vi "FisherPaykel Stop Motor.vi"(0 "VISA Refnum in":refnum<visa-resource-name>, 1 "Debug":bool, 2 "Use GEA Inverter Output":bool, 5 "Main Command":T2=">STP", 7 "GEA2 Reference In":refnum<k24>, 11 "Error In":errorcluster, 12 "GEA Stop Toggle":u8 max=1 step=1, 14 "GEA Inputs":T1={"Source"=228, "Destination"=35} {"Destination" format="%.0x"; "Source" format="%.0x"}) -> (4 "VISA Refnum out":refnum<visa-resource-name>, 6 "Command (Debug)":string, 8 "GEA2 Reference Out":refnum<k24>, 10 "GEA Stop Toggle Out":u8, 15 "Error Out":errorcluster)   [LabVIEW 2016]
uses:
  Type Definitions/Fisher Paykel Main Command.ctl
  Trunk/Utility/LabVIEW GEA2 Toolkit v1.0.0.0/type defs/Source_Destination.ctl
  C:/Technology Lab/NI-2010/Trunk/Utility/LabVIEW GEA2 Toolkit v1.0.0.0/Appliance.NET/GeaCommunication.dll
  Trunk/Utility/LabVIEW GEA2 Toolkit v1.0.0.0/Appliance.NET/GeaCommunication.dll
  Trunk/Utility/LabVIEW GEA2 Toolkit v1.0.0.0/type defs/ERD Write Data In.ctl
  Trunk/Utility/LabVIEW GEA2 Toolkit v1.0.0.0/type defs/Data Type.ctl
  Trunk/Utility/LabVIEW GEA2 Toolkit v1.0.0.0/library/GEA2_Toolkit.lvlib
panel:
  # "F&P Serial Commands"
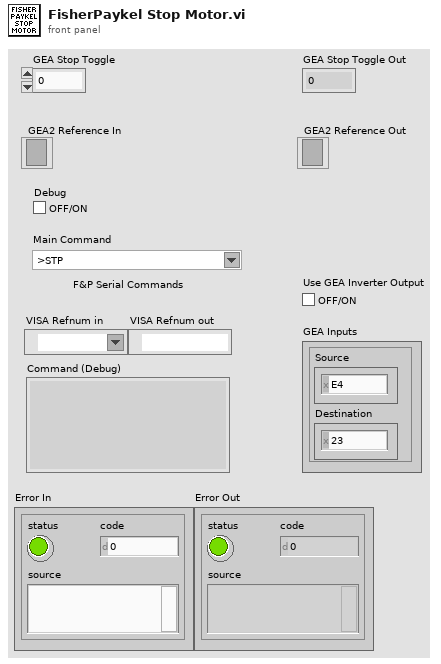
[diagram p1: front panel]
types:
  T1 = typedef "GEA2_Toolkit.lvlib/Source_Destination.ctl" = cluster{"Source":u8, "Destination":u8}
  T2 = typedef "Fisher Paykel Main Command.ctl" = string
  T3 = typedef "GEA2_Toolkit.lvlib/ERD Write Data In.ctl" = cluster{"ERD Number":u16, "Data Type":T4, "Data":string}
  T4 = typedef "GEA2_Toolkit.lvlib/Data Type.ctl" = enum16{"string", "boolean", "uint8_t", "uint16_t", "uint32_t", "uint64_t"}
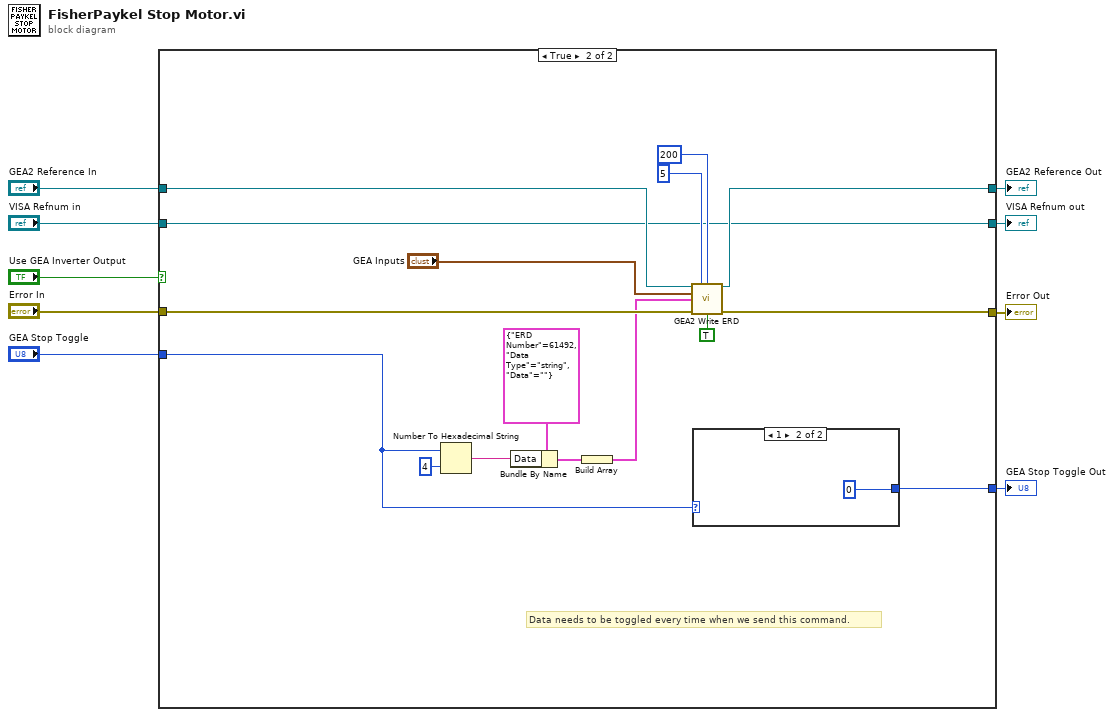
[diagram p0: block diagram]
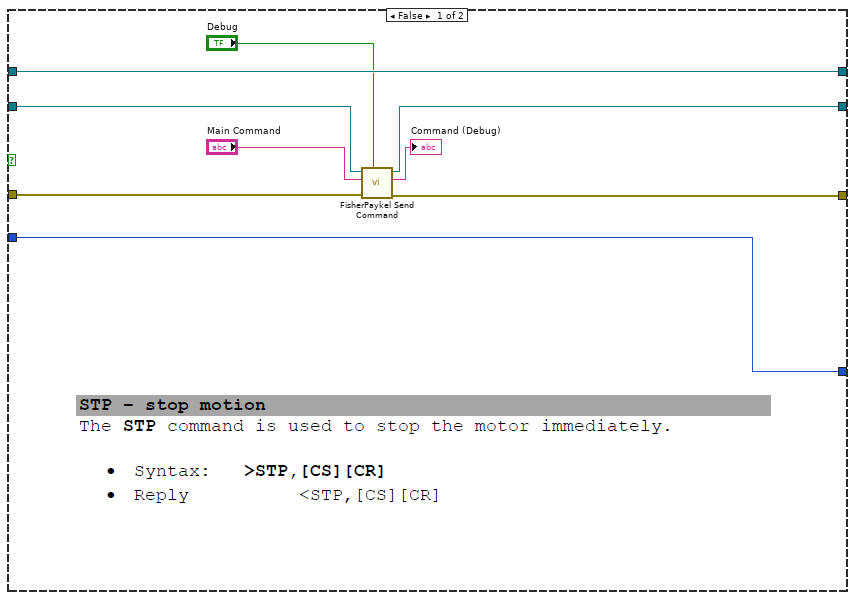
[diagram p2: hidden frame]
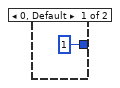
[diagram p3: hidden frame]
diagram:
  n1 = case shown="True" "Use GEA Inverter Output" {
    tunnel: [w17 w29] -> w9
    tunnel: "Error In" -> [w16 w30]
    tunnel: "VISA Refnum in" -> [w14 w26]
    tunnel: [w13 w26] -> w5
    tunnel: "GEA2 Reference In" -> [w12 w28]
    tunnel: [w12 w27] -> w3
    tunnel: "GEA Stop Toggle" -> [w10 w20]
    tunnel: [w10 w19] -> w1
    frame False {
      n2 = call "FisherPaykel Send Command.vi"("Debug"="Debug", "error in (no error)"=w16, "Send Command"="Main Command", "VISA Refnum in"=w14) -> ("error out"=w17:errorcluster, "Command (Debug)"=→"Command (Debug)":string, "VISA Refnum out"=w13:refnum<visa-resource-name>)  [unwired: 5 in]
    }
    frame True {
      # "Data needs to be toggled every time when we send this command."
      n3 = Number To Hexadecimal String(1:i16 4 ("width (-)"), 2:w20) -> (0:w25:string)
      n4 = Bundle By Name(cluster=T3 {"ERD Number"=61492, "Data Type"=enum."string", "Data"=""} ("ERD Write Data In"), "Data"=w25) -> (w23:T3)
      n5 = Build Array(w23) -> (w21:T3[])
      n6 = call "GEA2 Write ERD.vi"("GEA2 Reference In"=w28, "Retry Count"=5, "Read Timeout (ms)"=u32 200, "GEA Inputs"="GEA Inputs", "Write ERD List"=w21, "Error In"=w30, "Verify ERD Response?"=TRUE) -> ("GEA2 Reference Out"=w27:refnum<k24>, "Error Out"=w29:errorcluster)  [unwired: 6 in, 1 out]
      n7 = case shown="1" w20 {
        tunnel: [u8 1 ("GEA Stop Toggle 2") u8 0 ("GEA Stop Toggle 2")] -> w19
        frame 0, Default {
        }
        frame 1 {
        }
      }
    }
  }
  "Error Out" <- w9
  "VISA Refnum out" <- w5
  "GEA2 Reference Out" <- w3
  "GEA Stop Toggle Out" <- w1
